vi "set_params.vi"(8 "error in (no error)":errorcluster caption="entrée d'erreur (pas d'erreur)", 11 "SVC.lvclass 2":refnum<class "SVC.lvclass">) -> (0 "error out":errorcluster caption="sortie d'erreur", 3 "SVC.lvclass":refnum<class "SVC.lvclass">)   [LabVIEW 2020, in "SVC.lvclass"]
uses:
  SVC.lvclass
  SVC.lvclass/SVC.ctl
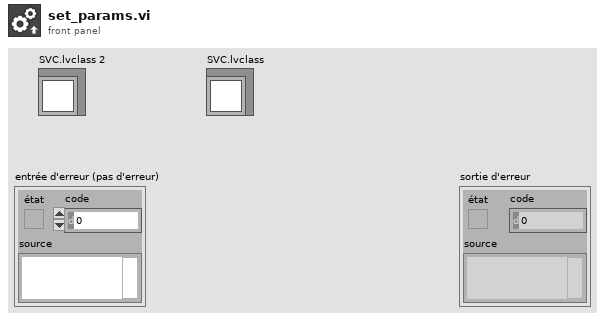
[diagram p1: front panel]
types:
  T1 = typedef "svc_params.ctl" = cluster{"C":dbl, "kernel":string, "degree":dbl, "gamma":cluster{"gamma_type":string, "gamma_float":dbl}, "coef0":dbl, "shrinking":bool, "probability":bool, "tol":dbl, "cache_size":dbl, "class_weight":cluster{"class_weight_type":string, "class_weight_dict":string}, "verbose":bool, "max_iter":dbl, "decision_function_shape":string, "break_ties":bool, "random_state":dbl}
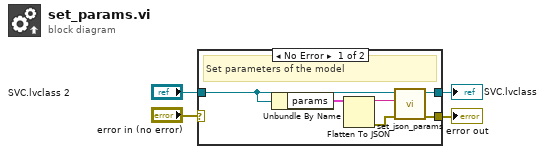
[diagram p0: block diagram]
diagram:
  n1 = case shown="No Error" "error in (no error)" {
    selector: "error in (no error)" -> [_ w12]
    tunnel: [w7 w12] -> w3
    tunnel: [w8 w11] -> w1
    tunnel: "SVC.lvclass 2" -> [w5 w11]
    frame No Error {
      # "Set parameters of the model"
      n2 = Unbundle By Name(w5) -> ("params"=w10:T1)
      n3 = Flatten To JSON(anything=w10) -> (JSON string=w9:string, 11:w6:errorcluster)  [unwired: 2 in]
      n4 = call-dynamic "set_json_params.vi"("error in (no error)"=w6, "params"=w9, "Model en entrée"=w5) -> ("error out"=w7:errorcluster, "Model en sortie"=w8:refnum<class "SVC.lvclass">)  [unwired: 7 in]
    }
    frame Error {
    }
  }
  "error out" <- w3
  "SVC.lvclass" <- w1
